vi "温度采集.vi"() -> ()   [LabVIEW 2020]
uses:
  <vilib>/Utility/file.llb/Write Delimited Spreadsheet (DBL).vi
  <vilib>/ptbypt/NI_PtbyPt.lvlib
panel:
  out "温度趋势图":cluster{"温度上限设定":dbl, dbl, "温度下限设定":dbl}(graph)
  out "报警灯":bool
  out "当前温度":dbl(slide) scale=0.0..100.0
  in  "温度下限设定":dbl format="%#_13g"
  in  "温度上限设定":dbl format="%#_13g"
  out "超越点数":dbl
  in  "通道切换":bool
  out "采样点数":i32
  in  "stop":bool
  out "mean":dbl caption="均值" format="%0.2f"
  out "min value":dbl caption="最小值" format="%0.2f"
  out "max value":dbl caption="最大值" format="%0.2f"
  # "ACH0"
  # "ACH1"
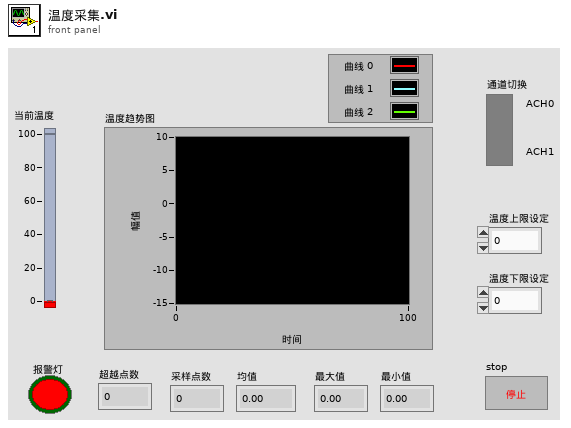
[diagram p1: front panel]
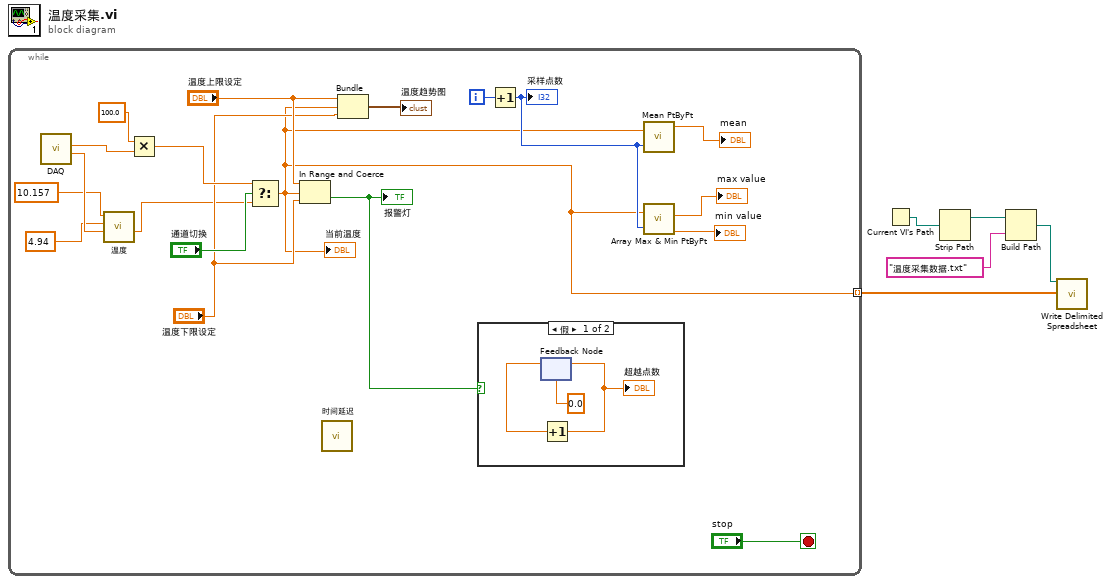
[diagram p0: block diagram]
diagram:
  n1 = while {
    tunnel: [w12] -> w1 mode=indexing
    i -> [w20]
    stop <- "stop" stop-if-true
    n2 = call "DAQ.vi"() -> ("Rt"=w9:dbl, "LM35"=w11:dbl)  [unwired: 10 in]
    n3 = call "温度.vi"("U"=w9, "Vcc"=4.94, "R"=10.157) -> ("Rt"=w10:dbl)  [unwired: 7 in, 1 out]
    n4 = Multiply(x=100.0, y=w11) -> (x*y=w19:dbl)
    n5 = Select(t=w19, s="通道切换", f=w10) -> (s? t:f=w12:dbl)
    "当前温度" <- w12
    n6 = In Range and Coerce(upper limit="温度上限设定", x=w12, lower limit="温度下限设定") -> (In Range?=w14:bool)  [unwired: 1 out]
    "报警灯" <- w14
    n7 = call "时间延迟"() -> ()  [unwired: 11 in, 1 out]
    n8 = Bundle("温度上限设定"="温度上限设定", "Rt"=w12, "温度下限设定"="温度下限设定") -> (→"温度趋势图":cluster{"温度上限设定":dbl, "Rt":dbl, "温度下限设定":dbl})  [unwired: 1 in]
    n9 = case shown="假" w14 {
      frame False {
        n10 = feedback #1(0.0) -> (w26:dbl)
        n11 = Increment(x=w26) -> (x+1=w27:dbl)
        "超越点数" <- w27
        n12 = feedback-in #1(w27) -> ()
      }
      frame True {
      }
    }
    n13 = Increment(x=w20) -> (x+1=w17:i32)
    "采样点数" <- w17
    n14 = call <vilib>:"Mean PtByPt.vi"("x"=w12, "sample length"=w17) -> ("mean"=→"mean":dbl)  [unwired: 2 in, 1 out]
    n15 = call <vilib>:"Array Max & Min PtByPt.vi"("input data point"=w12, "sample length"=w17) -> ("max value"=→"max value":dbl, "min value"=→"min value":dbl)  [unwired: 1 in, 3 out]
  }
  n16 = Current VI's Path() -> (path=w3:path)
  n17 = Strip Path(path=w3) -> (stripped path=w5:path)  [unwired: 1 out]
  n18 = Build Path(base path=w5, name or relative path="温度采集数据.txt") -> (appended path=w2:path)
  n19 = call-poly <vilib>:"Write Delimited Spreadsheet.vi"("file path (dialog if empty)"=w2, "1D data"=w1) -> ()  [unwired: 12 in, 2 out]
